vi "Get String DVR.vi"(8 "Error In":errorcluster, 11 "Pixel In":refnum<class "String.lvclass">) -> (0 "Error Out":errorcluster, 2 "DVR":refnum<data-value>, 3 "Pixel Out":refnum<class "String.lvclass">)   [LabVIEW 2019, in "String.lvclass"]
uses:
  String.lvclass
  Display Utilities/Display Utilities.lvlib
  Controls/Data.ctl
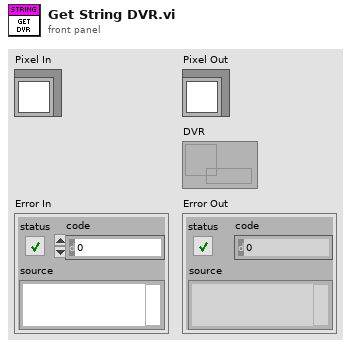
[diagram p1: front panel]
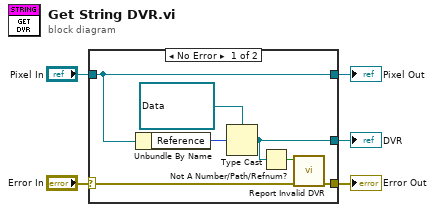
[diagram p0: block diagram]
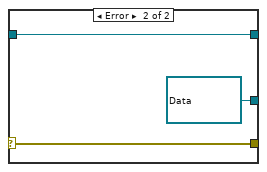
[diagram p2: hidden frame]
diagram:
  n1 = case shown="No Error" "Error In" {
    selector: "Error In" -> [w7 w15]
    tunnel: "Pixel In" -> [w11 w14]
    tunnel: [w6 w15] -> w4
    tunnel: [w11 w14] -> w2
    tunnel: [w9 refnum<data-value> refnum ("data value reference")] -> w1
    frame No Error {
      n2 = Unbundle By Name(w11) -> ("Reference"=w12:u64)
      n3 = Type Cast(type=refnum<data-value> refnum ("data value reference"), x=w12) -> (*(type *) &x=w9:refnum<data-value>)
      n4 = Not A Number/Path/Refnum?(number/path/refnum=w9) -> (NaN/Path/Refnum?=w8:bool)
      n5 = call "Report Invalid DVR.vi"("Error In"=w7, "Invalid DVR"=w8) -> ("Error Out"=w6:errorcluster)  [unwired: 9 in]
    }
    frame Error {
    }
  }
  "Error Out" <- w4
  "Pixel Out" <- w2
  "DVR" <- w1
